vi "Fdx Create Session (Tx-UDP Port-Oriented).vi"(6 "PortMap":u32, 8 "error in (no error)":errorcluster, 10 "port":u32, 11 "board":u32) -> (0 "error out":errorcluster, 2 "PortInitOut":T1 {"PortConfig" items=["FDX_SINGLE", "FDX_REDUNDANT"]}, 3 "port handle out":u32, 4 "Duplicated":bool, 5 "InstrumentHandle_board out":u32)   [LabVIEW 2020, in "AIM664LV.lvlib"]
uses:
  AIM664LV.lvlib
  _controls/hwEntry_actions.ctl
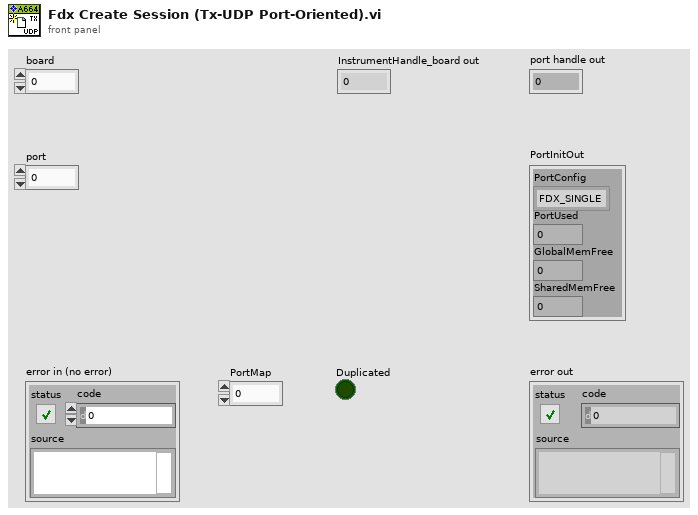
[diagram p1: front panel]
types:
  T1 = cluster{"PortConfig":u32, "PortUsed":u32, "GlobalMemFree":u32, "SharedMemFree":u32}
  T2 = typedef "AIM664LV.lvlib/hwEntry_actions.ctl" = enum16{"Init Port", "Init Board", "Relase Port", "Release Board"}
  T3 = typedef "AIM664LV.lvlib/hwEntry_handleValidityFlag.ctl" = cluster{"boardHandleValid":bool, "portHandleValid":bool}
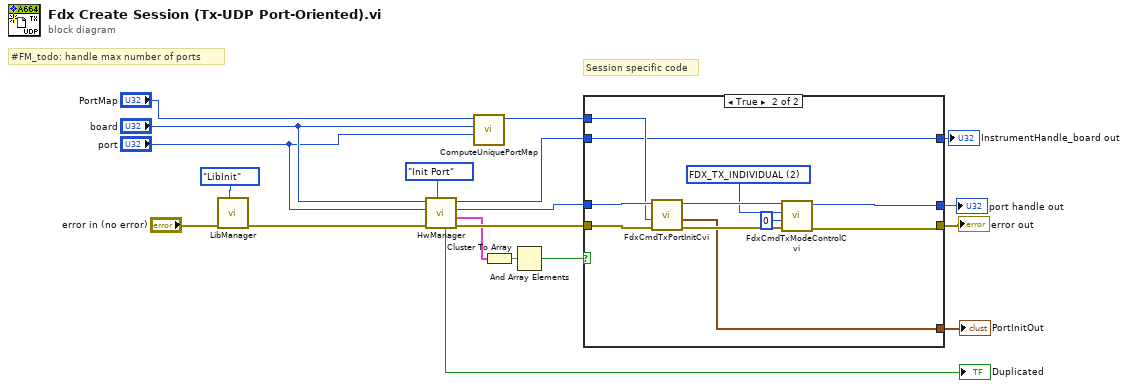
[diagram p0: block diagram]
diagram:
  # "Session specific code"
  # "#FM_todo: handle max number of ports"
  n1 = call "LibManager.vi"("action"=enum16{"LibInit", "LibExit"}."LibInit", "error in (no error)"="error in (no error)") -> ("error out"=w17:errorcluster)  [unwired: 7 in, 2 out]
  n2 = call "HwManager.vi"("action (Init)"=hwEntry_actions."Init Port", "error in (no error)"=w17, "port"="port", "board"="board") -> ("error out"=w16:errorcluster, "validityFlag"=w2:T3, "InstrumentHandle_port out"=w10:u32, "InstrumentHandle_board out"=w11:u32, "Duplicated"=→"Duplicated":bool)  [unwired: 3 in]
  n3 = call "ComputeUniquePortMap.vi"("port"="port", "board"="board", "PortMap In"="PortMap") -> ("PortMap out"=w13:u32)  [unwired: 8 in]
  n4 = Cluster To Array(cluster=w2) -> (array=w3:bool[])
  n5 = And Array Elements(Boolean array=w3) -> (logical AND=w1:bool)
  n6 = case shown="True" w1 {
    tunnel: w16 -> [w20 w29]
    tunnel: w10 -> [_ w25]
    tunnel: [w20 w26] -> w15
    tunnel: [_ w27] -> w14
    tunnel: w11 -> [_ w21]
    tunnel: w13 -> [_ w23]
    tunnel: [_ w22] -> w5
    tunnel: [_ w21] -> w4
    frame False {
    }
    frame True {
      w24 = u32 2 items=["FDX_TX_GENERIC", "FDX_TX_REPLAY", "FDX_TX_INDIVIDUAL"] ("TransmitMode")
      n7 = call "FdxCmdTxPortInitCvi.vi"("error in"=w29, "PortMap"=w23, "InstrumentHandle_port"=w25) -> ("error out"=w31:errorcluster, "PortInitOut"=w27:T1, "InstrumentHandle_port"=w28:u32)  [unwired: 6 in]
      n8 = call "FdxCmdTxModeControlCvi.vi"("error in"=w31, "RerosPortDelay"=u32 0, "TransmitMode"=w24, "InstrumentHandle_port"=w28) -> ("error out"=w26:errorcluster, "InstrumentHandle_port"=w22:u32)  [unwired: 6 in]
    }
  }
  "error out" <- w15
  "PortInitOut" <- w14
  "port handle out" <- w5
  "InstrumentHandle_board out" <- w4
